vi "Command Robot.vi"(11 "all rows":dbl[][](array[numeric])) -> ()   [LabVIEW 2020]
uses:
  Framework/Robot Global Data.vi
panel:
  out "Intake Sped Up":bool
  out "Transfer Release":bool
  out "Intake Reverse":bool
  out "Wheel":dbl
  out "Throttle":dbl
  out "Intake Arm Down":bool
  out "Intake Arm Up":bool
  out "Intake":bool
  out "Shooter":bool
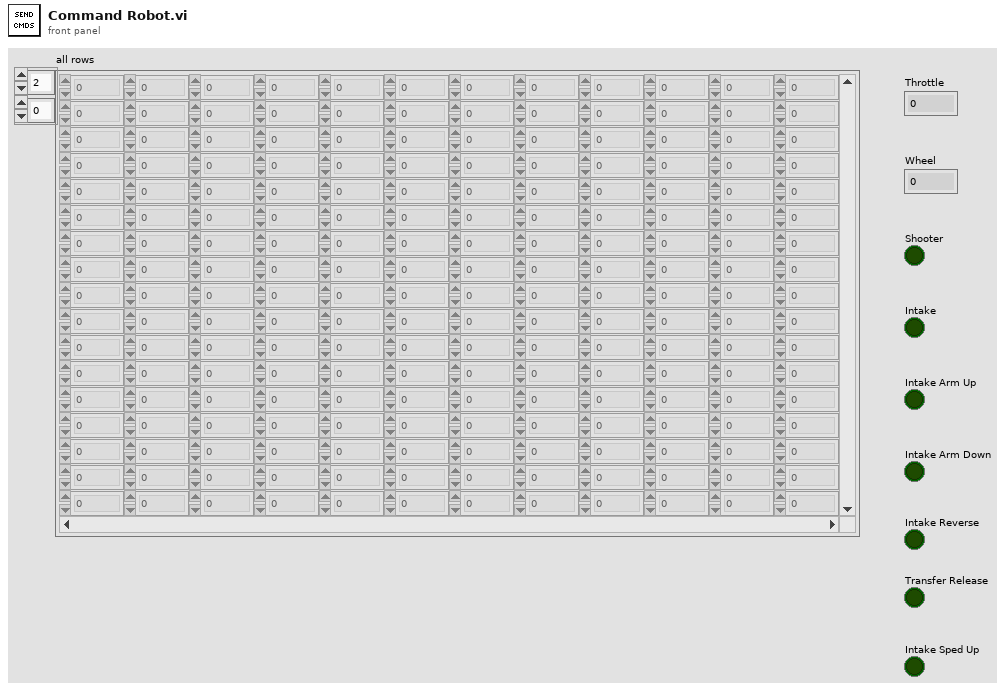
[diagram p1: front panel]
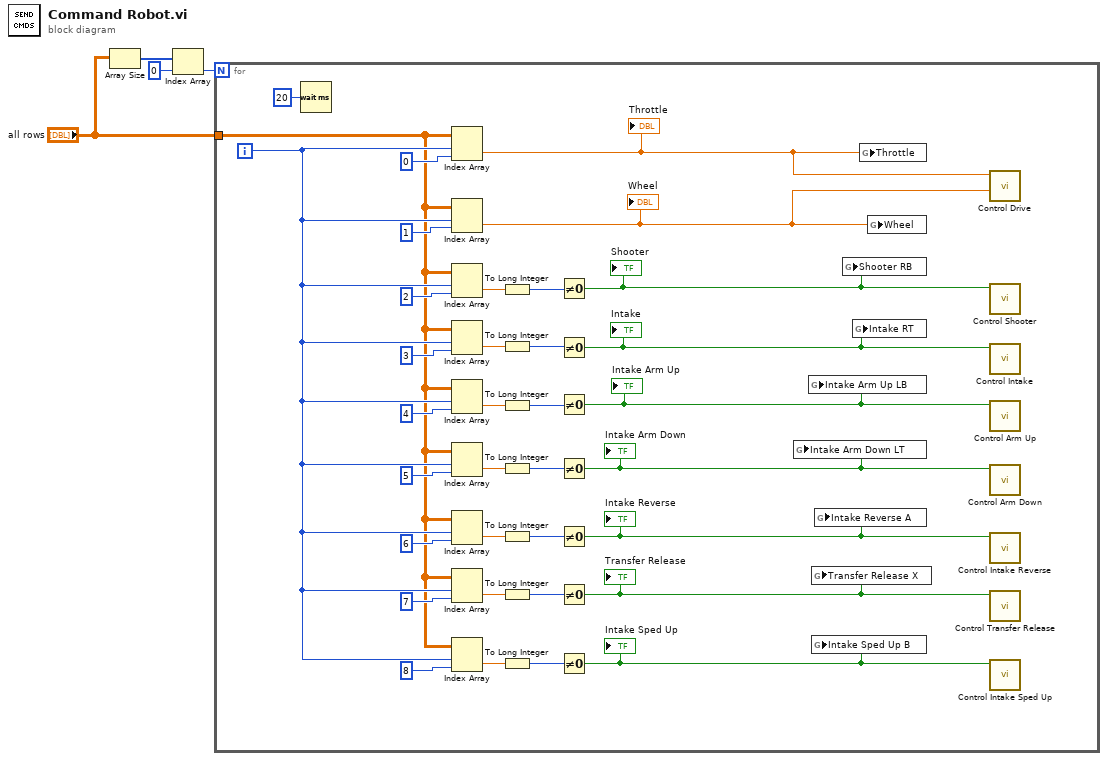
[diagram p0: block diagram]
diagram:
  n1 = Array Size(array="all rows") -> (size(s)=w2:i32[])
  n2 = Index Array(array=w2, index=0) -> (element=w1:i32)
  n3 = for {
    N: w1 -> [_]
    tunnel: "all rows" -> [w5]
    i -> [w6]
    n4 = Wait (ms)(milliseconds to wait=u32 20) -> ()  [unwired: 1 out]
    n5 = Index Array(array=w5, index (row)=w6, index (col)=0 ("disabled index (col)")) -> (element=w23:dbl)
    "Throttle" <- w23
    n6 = Index Array(array=w5, index (row)=w6, index (col)=1 ("disabled index (col)")) -> (element=w24:dbl)
    "Wheel" <- w24
    n7 = Index Array(array=w5, index (row)=w6, index (col)=2 ("disabled index (col)")) -> (element=w33:dbl)
    n8 = Index Array(array=w5, index (row)=w6, index (col)=3 ("disabled index (col)")) -> (element=w35:dbl)
    n9 = Index Array(array=w5, index (row)=w6, index (col)=4 ("disabled index (col)")) -> (element=w37:dbl)
    n10 = Index Array(array=w5, index (row)=w6, index (col)=5 ("disabled index (col)")) -> (element=w39:dbl)
    n11 = Index Array(array=w5, index (row)=w6, index (col)=6 ("disabled index (col)")) -> (element=w15:dbl)
    n12 = Index Array(array=w5, index (row)=w6, index (col)=7 ("disabled index (col)")) -> (element=w14:dbl)
    n13 = Index Array(array=w5, index (row)=w6, index (col)=8 ("disabled index (col)")) -> (element=w7:dbl)
    n14 = To Long Integer(number=w33) -> (32bit integer=w29:i32)
    n15 = To Long Integer(number=w35) -> (32bit integer=w28:i32)
    n16 = To Long Integer(number=w37) -> (32bit integer=w27:i32)
    n17 = To Long Integer(number=w39) -> (32bit integer=w26:i32)
    n18 = To Long Integer(number=w15) -> (32bit integer=w17:i32)
    n19 = To Long Integer(number=w14) -> (32bit integer=w12:i32)
    n20 = To Long Integer(number=w7) -> (32bit integer=w9:i32)
    n21 = Not Equal To 0?(x=w29) -> (x != 0?=w22:bool)
    "Shooter" <- w22
    n22 = Not Equal To 0?(x=w28) -> (x != 0?=w21:bool)
    "Intake" <- w21
    n23 = Not Equal To 0?(x=w27) -> (x != 0?=w20:bool)
    "Intake Arm Up" <- w20
    n24 = Not Equal To 0?(x=w26) -> (x != 0?=w19:bool)
    "Intake Arm Down" <- w19
    n25 = Not Equal To 0?(x=w17) -> (x != 0?=w18:bool)
    "Intake Reverse" <- w18
    n26 = Not Equal To 0?(x=w12) -> (x != 0?=w11:bool)
    "Transfer Release" <- w11
    n27 = Not Equal To 0?(x=w9) -> (x != 0?=w10:bool)
    "Intake Sped Up" <- w10
    n28 = global write "Robot Global Data.vi" "Intake Arm Down LT"(w19) -> ()
    n29 = global write "Robot Global Data.vi" "Intake Arm Up LB"(w20) -> ()
    n30 = global write "Robot Global Data.vi" "Transfer Release X"(w11) -> ()
    n31 = global write "Robot Global Data.vi" "Intake Sped Up B"(w10) -> ()
    n32 = global write "Robot Global Data.vi" "Intake Reverse A"(w18) -> ()
    n33 = global write "Robot Global Data.vi" "Shooter RB"(w22) -> ()
    n34 = global write "Robot Global Data.vi" "Intake RT"(w21) -> ()
    n35 = global write "Robot Global Data.vi" "Throttle"(w23) -> ()
    n36 = global write "Robot Global Data.vi" "Wheel"(w24) -> ()
    n37 = call "Control Drive.vi"("X-DriveAuto"=w24, "Y-DriveAuto"=w23) -> ()  [unwired: 10 in]
    n38 = call "Control Shooter.vi"("Avoid Race Condition"=w22) -> ()  [unwired: 11 in]
    n39 = call "Control Intake.vi"("Avoid Race Condition"=w21) -> ()  [unwired: 11 in]
    n40 = call "Control Arm Up.vi"("Avoid Race Condition"=w20) -> ()  [unwired: 11 in]
    n41 = call "Control Arm Down.vi"("Avoid Race Condition"=w19) -> ()  [unwired: 11 in]
    n42 = call "Control Intake Reverse.vi"("Avoid Race Condition"=w18) -> ()  [unwired: 11 in]
    n43 = call "Control Transfer Release.vi"("Avoid Race Condition"=w11) -> ()  [unwired: 11 in]
    n44 = call "Control Intake Sped Up.vi"("Avoid Race Condition"=w10) -> ()  [unwired: 11 in]
  }
